vi "afslag_minder (SubVI).vi"(11 "OK Button":bool) -> (3 "Numeric":dbl)   [LabVIEW 2019]
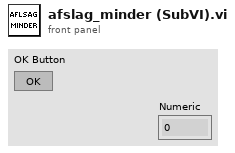
[diagram p1: front panel]
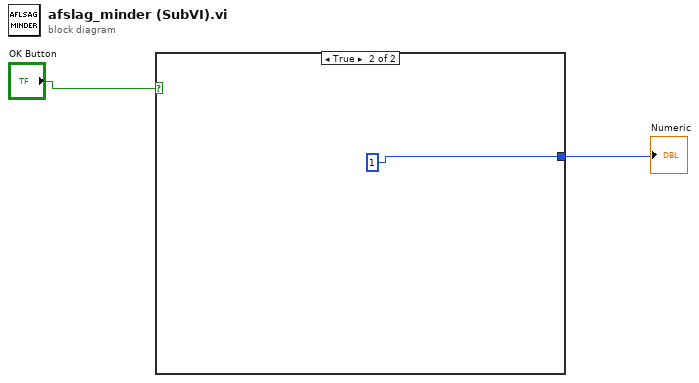
[diagram p0: block diagram]
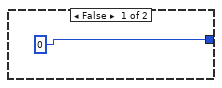
[diagram p2: hidden frame]
diagram:
  n1 = case shown="True" "OK Button" {
    tunnel: [0 1] -> w1
    frame False {
    }
    frame True {
    }
  }
  "Numeric" <- w1
